vi "MDPtrMgr GlobalSettings.vi"   [LabVIEW 2017, in "MDPtr.lvlib"]
uses:
  MDPtr.lvlib
  _MDPtrMgr/MDPtrMgr.lvclass
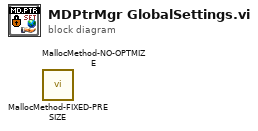
[diagram p0: block diagram]
diagram:
  n1 = call "MallocMethod-FIXED-PRESIZE.vi"() -> ()  [unwired: 11 in, 1 out]
  n2 = call "MallocMethod-NO-OPTMIZE.VI"() -> ()  [unwired: 11 in, 1 out]
